vi "Camera_Crop_Y_Axis.vi"(8 "Camera":T1, 10 "Detect Movement":bool, 11 "input cluster":T2 {"SystemVersion" items=["Standard", "XL"]; "Overlay_Ring" items=["Session Data", "Extended Setup", "Buffer", "Camera", "Dispenser", "Stats", "Connections"]; "Flush Size" min=1; "Dispense Speed" min=1; "Rectangle 2"."Rotation" format="%.2f"; "Rectangle 2"."Left" scale=0.0..1024.0; "Rectangle 2"."Right" scale=0.0..1024.0; "Rectangle 1"."Rotation" format="%.2f"; "Rectangle 1"."Left" scale=0.0..1024.0; "Rectangle 1"."Right" scale=0.0..1024.0; "Max Framerate" min=1; "Overload threshold" min=1; "Image Save Queue Size" min=1; "Image Process Queue Size" min=1; "Empty start" min=1; "Sample size threshold" min=1; "Framerate" min=1; "Light intensity" scale=0.0..100.0}) -> (1 "Height":i64, 3 "OffsetY":i64)   [LabVIEW 2022 SP3]
uses:
  controls/Data.ctl
  <vilib>/userdefined/High Color/IMAQdx.ctl
  <vilib>/vision/Image Controls.llb/IMAQ Image.ctl
  Camera_ID.ctl
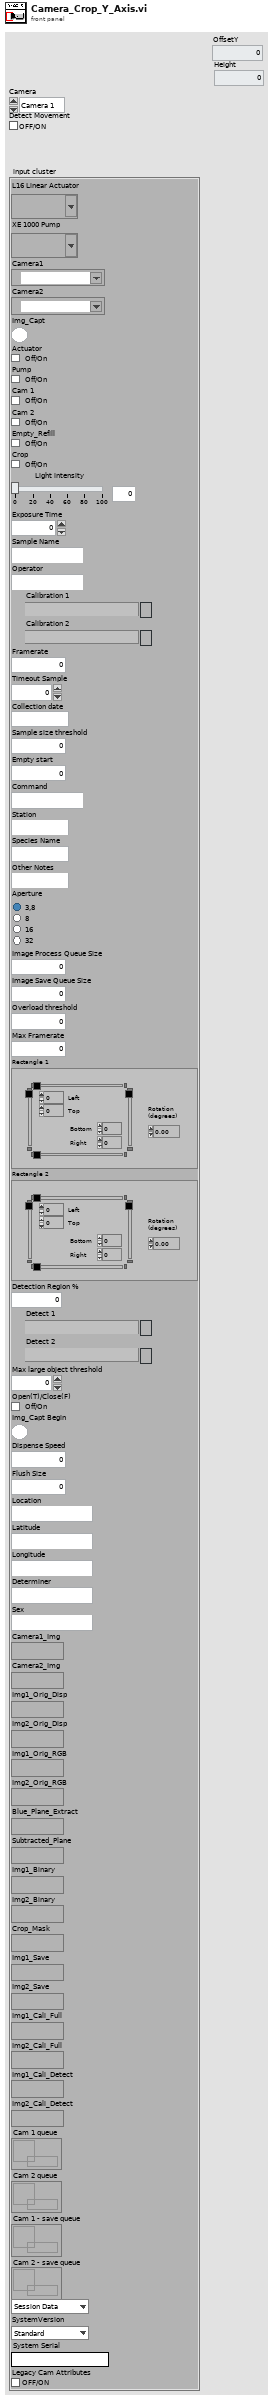
[diagram p1: front panel]
types:
  T1 = typedef "Camera_ID.ctl" = enum16{"Camera 1", "Camera 2"}
  T2 = typedef "Data.ctl" = cluster{"L16 Linear Actuator":refnum<visa-resource-name>, "XE 1000 Pump":refnum<visa-resource-name>, "Camera1":T3, "Camera2":T3, "Img_Capt":bool, "Actuator":bool, "Pump":bool, "Cam 1":bool, "Cam 2":bool, "Empty_Refill":bool, "Crop":bool, "Light intensity":i32, "Exposure Time":dbl, "Sample Name":string, "Operator":string, "Calibration 1":path, "Calibration 2":path, "Framerate":i32, "Timeout Sample":i32, "Collection date":string, "Sample size threshold":i32, "Empty start":u32, "Command":string, "Station":string, "Species Name":string, "Other Notes":string, "Aperture":enum32{"Item 0", "Item 1", "Item 2", "Item 3"}, "Image Process Queue Size":i32, "Image Save Queue Size":i32, "Overload threshold":i32, "Max Framerate":i32, "Rectangle 1":T4, "Rectangle 2":T4, "Detection Region %":dbl, "Detect 1":path, "Detect 2":path, "Max large object threshold":i32, "Open(T)/Close(F)":bool, "Img_Capt Begin":bool, "Dispense Speed":i32, "Flush Size":i32, "Location":string, "Latitude":string, "Longitude":string, "Determiner":string, "Sex":string, "Camera1_Img":T5, "Camera2_Img":T5, "Img1_Orig_Disp":T5, "Img2_Orig_Disp":T5, "Img1_Orig_RGB":T5, "Img2_Orig_RGB":T5, "Blue_Plane_Extract":T5, "Subtracted_Plane":T5, "Img1_Binary":T5, "Img2_Binary":T5, "Crop_Mask":T5, "Img1_Save":T5, "Img2_Save":T5, "Img1_Cali_Full":T5, "Img2_Cali_Full":T5, "Img1_Cali_Detect":T5, "Img2_Cali_Detect":T5, "Cam 1 queue":refnum<queue>, "Cam 2 queue":refnum<queue>, "Cam 1 - save queue":refnum<queue>, "Cam 2 - save queue":refnum<queue>, "Overlay_Ring":u16, "SystemVersion":u16, "System Serial":string, "Legacy Cam Attributes":bool}
  T3 = typedef "IMAQdx.ctl" = refnum<k21>
  T4 = typedef "IMAQ Rectangle" = cluster{"Left":i32, "Top":i32, "Right":i32, "Bottom":i32, "Rotation":dbl}
  T5 = typedef "IMAQ Image.ctl" = refnum<image>
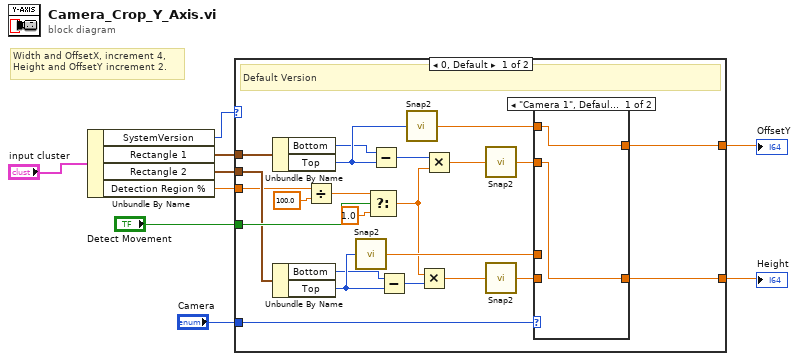
[diagram p0: block diagram]
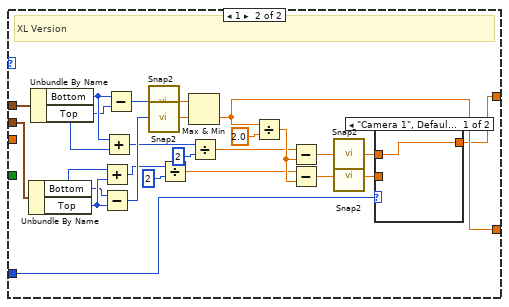
[diagram p3: hidden frame]
diagram:
  # "Width and OffsetX, increment 4,\nHeight and OffsetY increment 2."
  n1 = Unbundle By Name("input cluster") -> ("SystemVersion"=w1:u16, "Rectangle 1"=w6:T4, "Rectangle 2"=w7:T4, "Detection Region %"=w4:dbl)
  n2 = case shown="0, Default" w1 {
    tunnel: "Detect Movement" -> [w27 _]
    tunnel: w7 -> [w26 w42]
    tunnel: w6 -> [w25 w41]
    tunnel: "Camera" -> [w24 w43]
    tunnel: w4 -> [w19 _]
    tunnel: [w18 w45] -> w3
    tunnel: [w17 w44] -> w2
    frame 0, Default {
      # "Default Version"
      n3 = Unbundle By Name(w25) -> ("Bottom"=w14:i32, "Top"=w16:i32)
      n4 = Unbundle By Name(w26) -> ("Bottom"=w13:i32, "Top"=w15:i32)
      n5 = Divide(x=w19, y=100.0 ("x")) -> (x/y=w29:dbl)
      n6 = call "Snap2.vi"("x"=w15) -> ("x out"=w23:dbl)
      n7 = Select(t=w29, s=w27, f=1.0 ("t")) -> (s? t:f=w10:dbl)
      n8 = Subtract(x=w14, y=w16) -> (x-y=w31:i32)
      n9 = Subtract(x=w13, y=w15) -> (x-y=w32:i32)
      n10 = call "Snap2.vi"("x"=w16) -> ("x out"=w21:dbl)
      n11 = Multiply(x=w10, y=w32) -> (x*y=w11:dbl)
      n12 = Multiply(x=w31, y=w10) -> (x*y=w12:dbl)
      n13 = call "Snap2.vi"("x"=w12) -> ("x out"=w20:dbl)
      n14 = call "Snap2.vi"("x"=w11) -> ("x out"=w22:dbl)
      n15 = case shown="\"Camera 1\", Default" w24 {
        tunnel: w23 -> [_ w36]
        tunnel: [w34 w36] -> w17
        tunnel: w20 -> [w33 _]
        tunnel: [w33 w35] -> w18
        tunnel: w21 -> [w34 _]
        tunnel: w22 -> [_ w35]
        frame "Camera 1", Default {
        }
        frame "Camera 2" {
        }
      }
    }
    frame 1 {
      # "XL Version"
      n16 = Unbundle By Name(w42) -> ("Bottom"=w37:i32, "Top"=w38:i32)
      n17 = Unbundle By Name(w41) -> ("Bottom"=w40:i32, "Top"=w39:i32)
      n18 = Add(x=w37, y=w38) -> (x+y=w52:i32)
      n19 = Subtract(x=w37, y=w38) -> (x-y=w59:i32)
      n20 = Add(x=w40, y=w39) -> (x+y=w49:i32)
      n21 = Subtract(x=w40, y=w39) -> (x-y=w56:i32)
      n22 = call "Snap2.vi"("x"=w56) -> ("x out"=w57:dbl)
      n23 = call "Snap2.vi"("x"=w59) -> ("x out"=w60:dbl)
      n24 = Divide(x=w52, y=2) -> (x/y=w54:dbl)
      n25 = Max & Min(x=w57, y=w60) -> (min(x,y)=w45:dbl)  [unwired: 1 out]
      n26 = Divide(x=w49, y=2) -> (x/y=w51:dbl)
      n27 = Divide(x=w45, y=2.0) -> (x/y=w55:dbl)
      n28 = Subtract(x=w51, y=w55) -> (x-y=w58:dbl)
      n29 = Subtract(x=w54, y=w55) -> (x-y=w61:dbl)
      n30 = call "Snap2.vi"("x"=w58) -> ("x out"=w47:dbl)
      n31 = call "Snap2.vi"("x"=w61) -> ("x out"=w46:dbl)
      n32 = case shown="\"Camera 1\", Default" w43 {
        tunnel: w47 -> [w62 _]
        tunnel: [w62 w63] -> w44
        tunnel: w46 -> [_ w63]
        frame "Camera 1", Default {
        }
        frame "Camera 2" {
        }
      }
    }
  }
  "OffsetY" <- w2
  "Height" <- w3
